vi "FreqC.Self-test.vi"(8 "error In":errorcluster, 11 "FreqC Session in":T1) -> (0 "error out":errorcluster, 2 "Self-Test Result Code":i32, 3 "FreqC Session out":T1)   [LabVIEW 2018]
uses:
  typedefs/FreqC.Session.ctl
  <instrlib>/Agilent 532XX Series/Agilent 532XX Series.lvlib
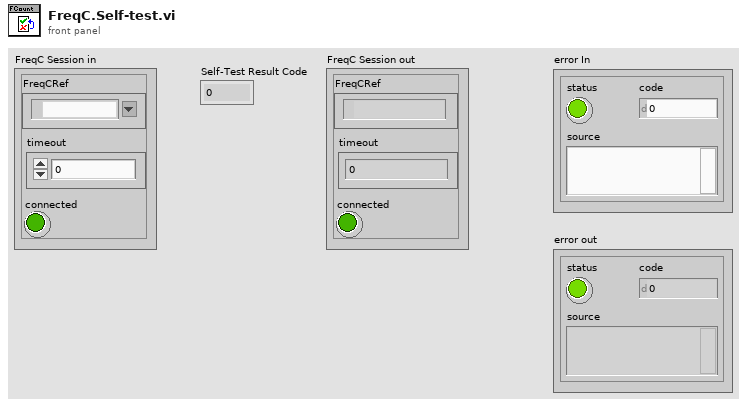
[diagram p1: front panel]
types:
  T1 = typedef "FreqC.Session.ctl" = cluster{"FreqCRef":refnum<visa-resource-name>, "timeout":dbl, "connected":bool}
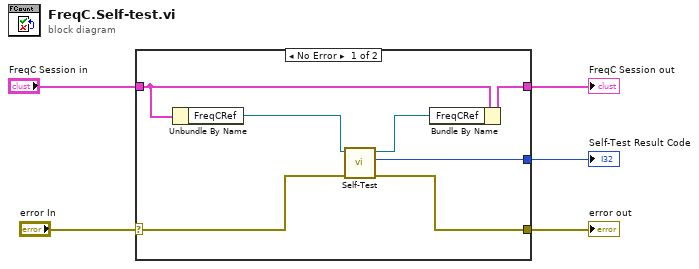
[diagram p0: block diagram]
diagram:
  n1 = case shown="No Error" "error In" {
    selector: "error In" -> [w8 w14]
    tunnel: [w7 w14] -> w4
    tunnel: "FreqC Session in" -> [w12 w13]
    tunnel: [w11 w13] -> w2
    tunnel: [w6 _] -> w1
    frame No Error {
      n2 = Unbundle By Name(w12) -> ("FreqCRef"=w10:refnum<visa-resource-name>)
      n3 = call <instrlib>:"Self-Test.vi"("error in (no error)"=w8, "VISA resource name"=w10) -> ("error out"=w7:errorcluster, "Self-Test Result Code"=w6:i32, "VISA resource name out"=w9:refnum<visa-resource-name>)  [unwired: 6 in, 1 out]
      n4 = Bundle By Name(cluster=w12, "FreqCRef"=w9) -> (w11:T1)
    }
    frame Error {
    }
  }
  "error out" <- w4
  "FreqC Session out" <- w2
  "Self-Test Result Code" <- w1
